vi "Drive to Image Height (Autonomous).vi"(1 "Execute":bool=TRUE, 2 "Image Height (Pixels)":dbl=10.0, 3 "Percent Velocity":dbl=0.8, 6 "Camera Stabilized?":bool) -> (4 "Done Executing":bool)   [LabVIEW 2012]
uses:
  Globals/Autonomous Joystick Emulation.vi
  Globals/Image Height.vi
  Globals/Alignment Error.vi
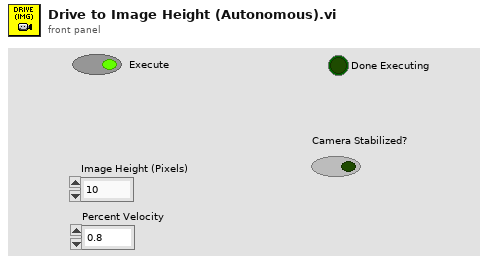
[diagram p1: front panel]
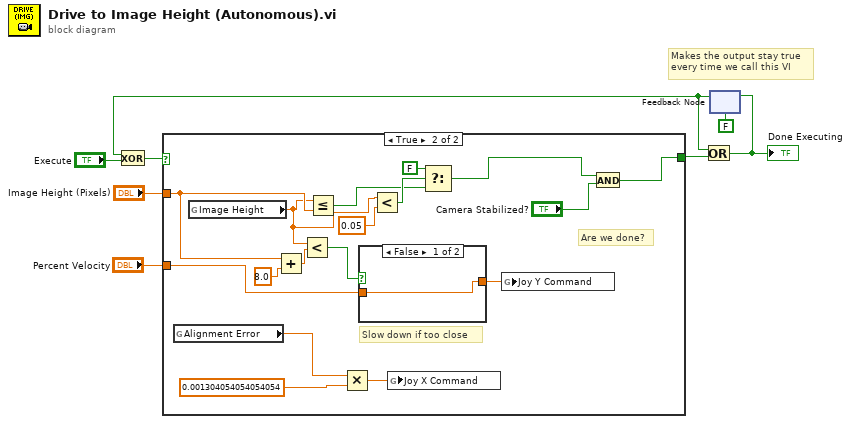
[diagram p0: block diagram]
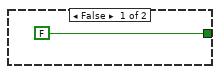
[diagram p2: hidden frame]
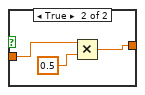
[diagram p3: hidden frame]
diagram:
  # "Makes the output stay true\nevery time we call this VI"
  n1 = feedback #1(FALSE) -> (w3:bool)
  n2 = Exclusive Or(1:"Execute", 2:w3) -> (0:w8:bool)
  n3 = case shown="True" w8 {
    tunnel: [FALSE w11] -> w6
    tunnel: "Percent Velocity" -> [_ w24]
    tunnel: "Image Height (Pixels)" -> [_ w18]
    frame False {
    }
    frame True {
      # "Slow down if too close"
      # "Are we done?"
      n4 = global read "Alignment Error.vi" "Alignment Error"() -> (w20:dbl)
      n5 = global read "Image Height.vi" "Image Height"() -> (w13:dbl)
      n6 = Add(x=w18, y=8.0) -> (x+y=w22:dbl)
      n7 = Less?(x=w13, y=w22) -> (x < y?=w26:bool)
      n8 = Less Or Equal?(x=w13, y=w18) -> (x <= y?=w15:bool)
      n9 = Multiply(x=w20, y=0.001304054054054054 ("Proportional Gain (Alignment)")) -> (x*y=w19:dbl)
      n10 = case shown="False" w26 {
        tunnel: [w27 w28] -> w25
        tunnel: w24 -> [w27 w30]
        frame False {
        }
        frame True {
          n11 = Multiply(x=w30, y=0.5) -> (x*y=w28:dbl)
        }
      }
      n12 = Less?(x=w13, y=0.05) -> (x < y?=w16:bool)
      n13 = global write "Autonomous Joystick Emulation.vi" "Joy X Command"(w19) -> ()
      n14 = Select(t=FALSE, s=w16, f=w15) -> (s? t:f=w12:bool)
      n15 = global write "Autonomous Joystick Emulation.vi" "Joy Y Command"(w25) -> ()
      n16 = And(x=w12, y="Camera Stabilized?") -> (x .and. y?=w11:bool)
    }
  }
  n17 = Or(x=w3, y=w6) -> (x .or. y?=w2:bool)
  "Done Executing" <- w2
  n18 = feedback-in #1(w2) -> ()
